vi "GetChannelConfAll.vi"(8 "error in":errorcluster, 10 "Channel Num":u32, 11 "CAN-NI":refnum<class "CAN-NI.lvclass">) -> (0 "error out":errorcluster, 2 "ChannelProperty":T1, 3 "CAN-NI":refnum<class "CAN-NI.lvclass">)   [LabVIEW 2019, in "CAN-NI.lvlib" / "CAN-NI.lvclass"]
uses:
  CAN-NI.lvclass
  TypeDef/ChannelProperty.ctl
  CAN-Interface/TypeDef/Def-Termination.ctl
  CAN-Interface/TypeDef/Def-Transmit Mode.ctl
  CAN-Interface/TypeDef/Def-Protocol.ctl
  CAN-NI.lvclass/CAN-NI.ctl
  CAN-Interface/Class-Interface.lvclass
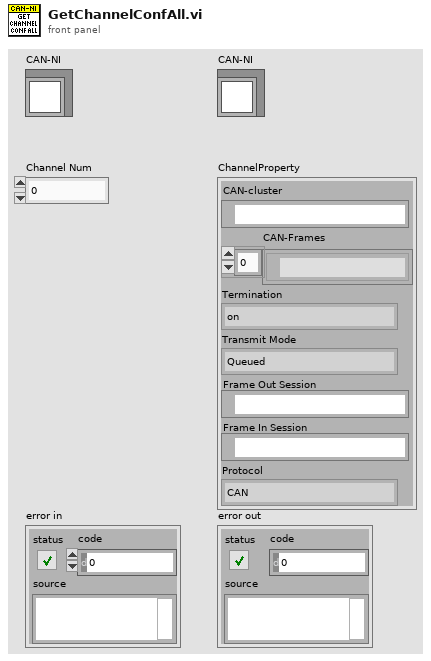
[diagram p1: front panel]
types:
  T1 = typedef "CAN-NI.lvlib/CAN-NI.lvclass/ChannelProperty.ctl" = cluster{"CAN-cluster":refnum<k21>, "CAN-Frames":refnum<k21>[], "Termination":T2, "Transmit Mode":T3, "Frame Out Session":refnum<k21>, "Frame In Session":refnum<k21>, "Protocol":T4}
  T2 = typedef "CAN-Interface.lvlib/Class-Interface.lvclass/Def-Termination.ctl" = enum8{"on", "off"}
  T3 = typedef "CAN-Interface.lvlib/Class-Interface.lvclass/Def-Transmit Mode.ctl" = enum16{"Queued", "Stream"}
  T4 = typedef "CAN-Interface.lvlib/Class-Interface.lvclass/Def-Protocol.ctl" = enum16{"CAN", "CAN FD"}
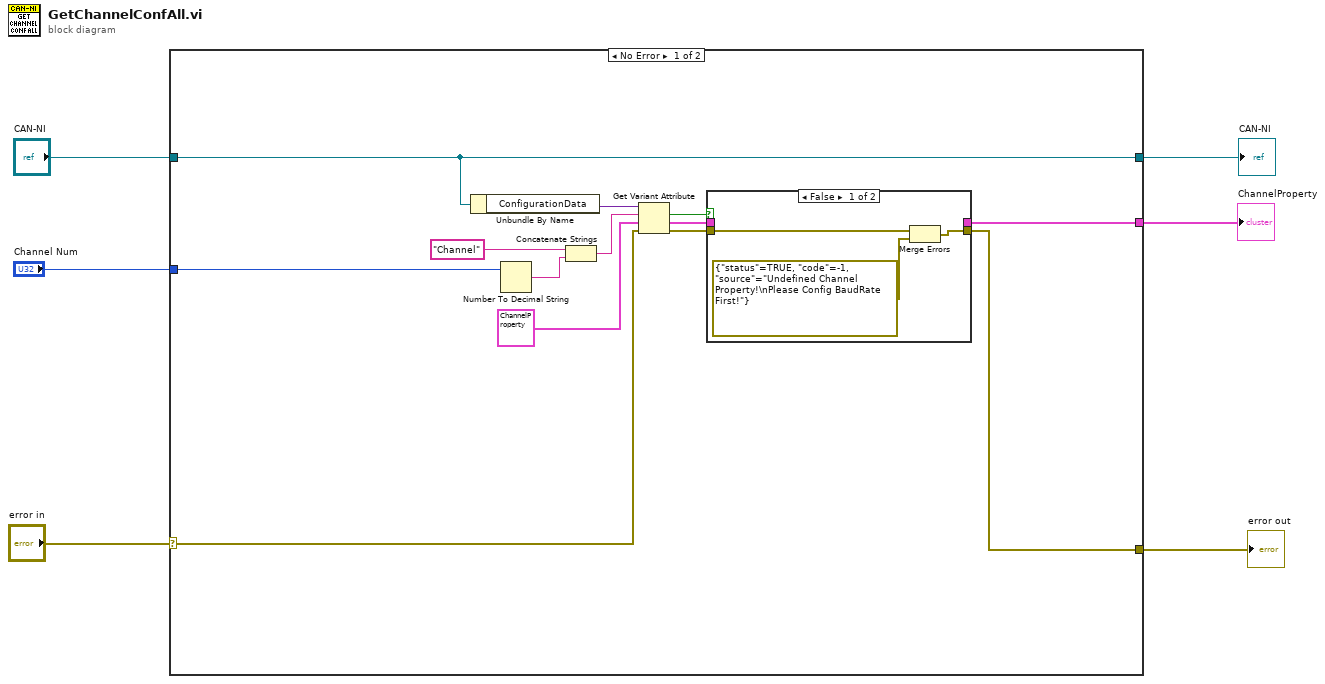
[diagram p0: block diagram]
diagram:
  n1 = case shown="No Error" "error in" {
    selector: "error in" -> [w10 w26]
    tunnel: "CAN-NI" -> [w7 w25]
    tunnel: "Channel Num" -> [w17 _]
    tunnel: [w11 _] -> w3
    tunnel: [w8 w26] -> w2
    tunnel: [w7 w25] -> w1
    frame No Error {
      n2 = Unbundle By Name(w7) -> ("ConfigurationData"=w16:variant)
      n3 = Number To Decimal String(number=w17) -> (decimal integer string=w19:string)  [unwired: 1 in]
      n4 = Concatenate Strings("Channel" ("string"), w19) -> (w15:string)
      n5 = Get Variant Attribute(Variant=w16, name=w15, default value (empty Variant)=T1 {"CAN-cluster"="", "CAN-Frames"=[], "Termination"=enum."on", "Transmit Mode"=enum."Queued", "Frame Out Session"="", "Frame In Session"="", "Protocol"=enum."CAN"} ("ChannelProperty"), error in=w10) -> (found=w13:bool, value=w12:T1, error out=w9:errorcluster)  [unwired: 1 out]
      n6 = case shown="False" w13 {
        tunnel: w12 -> [_ w24]
        tunnel: [_ w24] -> w11
        tunnel: w9 -> [w22 w23]
        tunnel: [w20 w23] -> w8
        frame False {
          n7 = Merge Errors(w22, errorcluster {"status"=TRUE, "code"=-1, "source"="Undefined Channel Property!\nPlease Config BaudRate First!"} ("error in (no error)")) -> (w20:errorcluster)
        }
        frame True {
        }
      }
    }
    frame Error {
    }
  }
  "ChannelProperty" <- w3
  "error out" <- w2
  "CAN-NI" <- w1
